vi "Compile Core.vi"(8 "error in (no error)":errorcluster, 10 "Compiled Data":T1 {"DI-B Injection"."Settings"."Pump Phase Array"."Profile" max=15; "DI-B Injection"."Settings"."Pump Phase Array"."Period [s]" min=0 max=0.000102 format="%#_3p"; "DI-B Injection"."Settings"."Pump Phase Array"."Pulse Width [s]" min=0 max=0.000102 format="%#_3p"; "DI-B Injection"."Settings"."Pump Phase Array"."Voltage Low [V]" min=-250 max=250 format="%#_3p"; "DI-B Injection"."Settings"."Pump Phase Array"."Voltage High [V]" min=-250 max=250 format="%#_3p"; "DI-B Injection"."Settings"."Pump Phase Array"."Current Low [A]" min=-40 max=40 format="%#_3p"; "DI-B Injection"."Settings"."Pump Phase Array"."Current High [A]" min=-40 max=40 format="%#_3p"; "DI-B Injection"."Settings"."Pump Phase Array"."Duration [s]" min=0 max=1.67772 format="%#_3p"; "DI-B Injection"."Settings"."Inj Phase Arrays"."Profile" max=15; "DI-B Injection"."Settings"."Inj Phase Arrays"."Period [s]" min=0 max=0.000102 format="%#_3p"; "DI-B Injection"."Settings"."Inj Phase Arrays"."Pulse Width [s]" min=0 max=0.000102 format="%#_3p"; "DI-B Injection"."Settings"."Inj Phase Arrays"."Voltage Low [V]" min=-250 max=250 format="%#_3p"; "DI-B Injection"."Settings"."Inj Phase Arrays"."Voltage High [V]" min=-250 max=250 format="%#_3p"; "DI-B Injection"."Settings"."Inj Phase Arrays"."Current Low [A]" min=-40 max=40 format="%#_3p"; "DI-B Injection"."Settings"."Inj Phase Arrays"."Current High [A]" min=-40 max=40 format="%#_3p"; "DI-B Injection"."Settings"."Inj Phase Arrays"."Duration [s]" min=0 max=1.67772 format="%#_3p"; "DI-A Injection"."Settings"."Pump Phase Array"."Profile" max=15; "DI-A Injection"."Settings"."Pump Phase Array"."Period [s]" min=0 max=0.000102 format="%#_3p"; "DI-A Injection"."Settings"."Pump Phase Array"."Pulse Width [s]" min=0 max=0.000102 format="%#_3p"; "DI-A Injection"."Settings"."Pump Phase Array"."Voltage Low [V]" min=-250 max=250 format="%#_3p"; "DI-A Injection"."Settings"."Pump Phase Array"."Voltage High [V]" min=-250 max=250 format="%#_3p"; "DI-A Injection"."Settings"."Pump Phase Array"."Current Low [A]" min=-40 max=40 format="%#_3p"; "DI-A Injection"."Settings"."Pump Phase Array"."Current High [A]" min=-40 max=40 format="%#_3p"; "DI-A Injection"."Settings"."Pump Phase Array"."Duration [s]" min=0 max=1.67772 format="%#_3p"; "DI-A Injection"."Settings"."Inj Phase Arrays"."Profile" max=15; "DI-A Injection"."Settings"."Inj Phase Arrays"."Period [s]" min=0 max=0.000102 format="%#_3p"; "DI-A Injection"."Settings"."Inj Phase Arrays"."Pulse Width [s]" min=0 max=0.000102 format="%#_3p"; "DI-A Injection"."Settings"."Inj Phase Arrays"."Voltage Low [V]" min=-250 max=250 format="%#_3p"; "DI-A Injection"."Settings"."Inj Phase Arrays"."Voltage High [V]" min=-250 max=250 format="%#_3p"; "DI-A Injection"."Settings"."Inj Phase Arrays"."Current Low [A]" min=-40 max=40 format="%#_3p"; "DI-A Injection"."Settings"."Inj Phase Arrays"."Current High [A]" min=-40 max=40 format="%#_3p"; "DI-A Injection"."Settings"."Inj Phase Arrays"."Duration [s]" min=0 max=1.67772 format="%#_3p"; "Knock"."Settings"."Sensor Select" items=["Sensor 1", "Sensor 2", "Sensor 3", "Sensor 4", "Sensor 5", "Sensor 6", "Sensor 7", "Sensor 8", "Sensor 9", "Sensor 10", "Sensor 11", "Sensor 12"]; "PBx"."PB-01"."FIFO Indexes"."Read"."UEGO Diagnostics"."LSUType" format="%02.0f"; "PBx"."PB-01"."FIFO Indexes"."Read"."UEGO Diagnostics"."UEGOFuseStatus" format="%02.0f"; "DCM Core"."Settings"."System Settings"."HH Open Threshold [A]" min=0 max=8 format="%#_3p"; "DCM Core"."Settings"."System Settings"."HH ISeq Dur PS" items=["3.3ms @ 20MHz"=0, "6.5ms @ 10MHz"=4, "13ms @ 5MHz"=6, "26ms @ 2.5MHz"=7]; "DCM Core"."Settings"."System Settings"."HH Shoot Through Time [s]" min=0 max=0.003277 format="%#_3p"; "DCM Core"."Settings"."System Settings"."Clamp Fault Filter Time [s]" min=0 max=0.003277 format="%#_3p"; "DCM Core"."Settings"."System Settings"."DI HS Fault Filter Time [s]" min=0 max=0.003277 format="%#_3p"; "DCM Core"."Settings"."B Configuration"."Pump Zener Voltage [V]" min=0 max=240 format="%#_13g"; "DCM Core"."Settings"."B Configuration"."DI Zener Voltage [V]" min=0 max=100 format="%#_13g"; "DCM Core"."Settings"."B Configuration"."Boost Clamp [V]" min=0 max=220 format="%#_13g"; "DCM Core"."Settings"."B Configuration"."Boost Voltage [V]" min=0 max=220 format="%#_13g"; "DCM Core"."Settings"."A Configuration"."Pump Zener Voltage [V]" min=0 max=240 format="%#_13g"; "DCM Core"."Settings"."A Configuration"."DI Zener Voltage [V]" min=0 max=100 format="%#_13g"; "DCM Core"."Settings"."A Configuration"."Boost Clamp [V]" min=0 max=220 format="%#_13g"; "DCM Core"."Settings"."A Configuration"."Boost Voltage [V]" min=0 max=220 format="%#_13g"; "DCM Core"."FIFO Indexes"."Write"."HH Config"."ISeq"."Duration [s]" min=0 max=26; "DCM Core"."FIFO Indexes"."Write"."HH Config"."ISeq"."Lower [A]" min=0 max=8; "DCM Core"."FIFO Indexes"."Write"."HH Config"."ISeq"."Upper [A]" min=0 max=8; "Digital Signals"."Settings"."Aux In Filters [s]" min=0; "Digital Signals"."Settings"."Diff IO Filters [s]" min=0; "EPTx RevA"."Settings"."EPTxFilters"."Aux 4 [s]" format="%#_6p"; "EPTx RevA"."Settings"."EPTxFilters"."Aux 3 [s]" format="%#_6p"; "EPTx RevA"."Settings"."EPTxFilters"."Aux 2 [s]" format="%#_6p"; "EPTx RevA"."Settings"."EPTxFilters"."Aux 1 [s]" format="%#_6p"; "EPTx RevA"."Settings"."EPTxFilters"."Primary [s]" format="%#_6p"}, 11 "Device Item Ref in":T40 format="%.0x") -> (0 "error out":errorcluster, 2 "Compiled Data":T1 {"DI-B Injection"."Settings"."Pump Phase Array"."Profile" max=15; "DI-B Injection"."Settings"."Pump Phase Array"."Period [s]" min=0 max=0.000102 format="%#_3p"; "DI-B Injection"."Settings"."Pump Phase Array"."Pulse Width [s]" min=0 max=0.000102 format="%#_3p"; "DI-B Injection"."Settings"."Pump Phase Array"."Voltage Low [V]" min=-250 max=250 format="%#_3p"; "DI-B Injection"."Settings"."Pump Phase Array"."Voltage High [V]" min=-250 max=250 format="%#_3p"; "DI-B Injection"."Settings"."Pump Phase Array"."Current Low [A]" min=-40 max=40 format="%#_3p"; "DI-B Injection"."Settings"."Pump Phase Array"."Current High [A]" min=-40 max=40 format="%#_3p"; "DI-B Injection"."Settings"."Pump Phase Array"."Duration [s]" min=0 max=1.67772 format="%#_3p"; "DI-B Injection"."Settings"."Inj Phase Arrays"."Profile" max=15; "DI-B Injection"."Settings"."Inj Phase Arrays"."Period [s]" min=0 max=0.000102 format="%#_3p"; "DI-B Injection"."Settings"."Inj Phase Arrays"."Pulse Width [s]" min=0 max=0.000102 format="%#_3p"; "DI-B Injection"."Settings"."Inj Phase Arrays"."Voltage Low [V]" min=-250 max=250 format="%#_3p"; "DI-B Injection"."Settings"."Inj Phase Arrays"."Voltage High [V]" min=-250 max=250 format="%#_3p"; "DI-B Injection"."Settings"."Inj Phase Arrays"."Current Low [A]" min=-40 max=40 format="%#_3p"; "DI-B Injection"."Settings"."Inj Phase Arrays"."Current High [A]" min=-40 max=40 format="%#_3p"; "DI-B Injection"."Settings"."Inj Phase Arrays"."Duration [s]" min=0 max=1.67772 format="%#_3p"; "DI-A Injection"."Settings"."Pump Phase Array"."Profile" max=15; "DI-A Injection"."Settings"."Pump Phase Array"."Period [s]" min=0 max=0.000102 format="%#_3p"; "DI-A Injection"."Settings"."Pump Phase Array"."Pulse Width [s]" min=0 max=0.000102 format="%#_3p"; "DI-A Injection"."Settings"."Pump Phase Array"."Voltage Low [V]" min=-250 max=250 format="%#_3p"; "DI-A Injection"."Settings"."Pump Phase Array"."Voltage High [V]" min=-250 max=250 format="%#_3p"; "DI-A Injection"."Settings"."Pump Phase Array"."Current Low [A]" min=-40 max=40 format="%#_3p"; "DI-A Injection"."Settings"."Pump Phase Array"."Current High [A]" min=-40 max=40 format="%#_3p"; "DI-A Injection"."Settings"."Pump Phase Array"."Duration [s]" min=0 max=1.67772 format="%#_3p"; "DI-A Injection"."Settings"."Inj Phase Arrays"."Profile" max=15; "DI-A Injection"."Settings"."Inj Phase Arrays"."Period [s]" min=0 max=0.000102 format="%#_3p"; "DI-A Injection"."Settings"."Inj Phase Arrays"."Pulse Width [s]" min=0 max=0.000102 format="%#_3p"; "DI-A Injection"."Settings"."Inj Phase Arrays"."Voltage Low [V]" min=-250 max=250 format="%#_3p"; "DI-A Injection"."Settings"."Inj Phase Arrays"."Voltage High [V]" min=-250 max=250 format="%#_3p"; "DI-A Injection"."Settings"."Inj Phase Arrays"."Current Low [A]" min=-40 max=40 format="%#_3p"; "DI-A Injection"."Settings"."Inj Phase Arrays"."Current High [A]" min=-40 max=40 format="%#_3p"; "DI-A Injection"."Settings"."Inj Phase Arrays"."Duration [s]" min=0 max=1.67772 format="%#_3p"; "Knock"."Settings"."Sensor Select" items=["Sensor 1", "Sensor 2", "Sensor 3", "Sensor 4", "Sensor 5", "Sensor 6", "Sensor 7", "Sensor 8", "Sensor 9", "Sensor 10", "Sensor 11", "Sensor 12"]; "PBx"."PB-01"."FIFO Indexes"."Read"."UEGO Diagnostics"."LSUType" format="%02.0f"; "PBx"."PB-01"."FIFO Indexes"."Read"."UEGO Diagnostics"."UEGOFuseStatus" format="%02.0f"; "DCM Core"."Settings"."System Settings"."HH Open Threshold [A]" min=0 max=8 format="%#_3p"; "DCM Core"."Settings"."System Settings"."HH ISeq Dur PS" items=["3.3ms @ 20MHz"=0, "6.5ms @ 10MHz"=4, "13ms @ 5MHz"=6, "26ms @ 2.5MHz"=7]; "DCM Core"."Settings"."System Settings"."HH Shoot Through Time [s]" min=0 max=0.003277 format="%#_3p"; "DCM Core"."Settings"."System Settings"."Clamp Fault Filter Time [s]" min=0 max=0.003277 format="%#_3p"; "DCM Core"."Settings"."System Settings"."DI HS Fault Filter Time [s]" min=0 max=0.003277 format="%#_3p"; "DCM Core"."Settings"."B Configuration"."Pump Zener Voltage [V]" min=0 max=240 format="%#_13g"; "DCM Core"."Settings"."B Configuration"."DI Zener Voltage [V]" min=0 max=100 format="%#_13g"; "DCM Core"."Settings"."B Configuration"."Boost Clamp [V]" min=0 max=220 format="%#_13g"; "DCM Core"."Settings"."B Configuration"."Boost Voltage [V]" min=0 max=220 format="%#_13g"; "DCM Core"."Settings"."A Configuration"."Pump Zener Voltage [V]" min=0 max=240 format="%#_13g"; "DCM Core"."Settings"."A Configuration"."DI Zener Voltage [V]" min=0 max=100 format="%#_13g"; "DCM Core"."Settings"."A Configuration"."Boost Clamp [V]" min=0 max=220 format="%#_13g"; "DCM Core"."Settings"."A Configuration"."Boost Voltage [V]" min=0 max=220 format="%#_13g"; "DCM Core"."FIFO Indexes"."Write"."HH Config"."ISeq"."Duration [s]" min=0 max=26; "DCM Core"."FIFO Indexes"."Write"."HH Config"."ISeq"."Lower [A]" min=0 max=8; "DCM Core"."FIFO Indexes"."Write"."HH Config"."ISeq"."Upper [A]" min=0 max=8; "Digital Signals"."Settings"."Aux In Filters [s]" min=0; "Digital Signals"."Settings"."Diff IO Filters [s]" min=0; "EPTx RevA"."Settings"."EPTxFilters"."Aux 4 [s]" format="%#_6p"; "EPTx RevA"."Settings"."EPTxFilters"."Aux 3 [s]" format="%#_6p"; "EPTx RevA"."Settings"."EPTxFilters"."Aux 2 [s]" format="%#_6p"; "EPTx RevA"."Settings"."EPTxFilters"."Aux 1 [s]" format="%#_6p"; "EPTx RevA"."Settings"."EPTxFilters"."Primary [s]" format="%#_6p"}, 3 "Device Item Ref out":T40 format="%.0x")   [LabVIEW 2016, in "DCM System Explorer.lvlib"]
uses:
  DCM System Explorer.lvlib
  <vilib>/NI Veristand/Custom Device API/Custom Device Item Ref.ctl
  Shared/Types/HH Config Indexes.ctl
  Shared/Types/HH Status Indexes.ctl
  Shared/Types/DI Faults Indexes.ctl
  Shared/Types/System State Indexes.ctl
  Shared/Types/Compiled Data.ctl
  <vilib>/NI Veristand/Custom Device Waveform API/Multiple Waveforms Write (DBL)/Multiple Waveforms Write (DBL).lvclass
  Shared/Types/Engine Init Data.ctl
  Shared/Types/Engine Status.ctl
  Shared/Types/EPTx RevA RT Data.ctl
  Built/DCM Classes Packed/Pharlap/C/DCM-Classes.lvlibp/1abvi3w/vi.lib/Powertrain Controls/Device Drivers/DCM/Rev0/FPGA/Digital Channel.ctl
  Built/DCM Classes Packed/Pharlap/C/DCM-Classes.lvlibp/Engine Position Tracking/EPTx/RevA/RT/Controls/EPTxFilters.ctl
  Shared/Types/DCM Core.ctl
  <vilib>/Powertrain Controls/Device Drivers/DCM/Rev0/RT/Configuration.ctl
  <vilib>/Powertrain Controls/Device Drivers/DCM/Rev0/FPGA/DI - Bank Configuration.ctl
  <vilib>/Powertrain Controls/Device Drivers/DCM/Rev0/RT/System Settings.ctl
  <vilib>/Powertrain Controls/Device Drivers/DCM/Rev0/RT/User LED.ctl
  <vilib>/Powertrain Controls/Device Drivers/DCM/HH/RT/Duration Pre Scale.ctl
  Shared/Types/DI.ctl
  Shared/Types/DI Command Indexes.ctl
  Shared/Types/DI Phase Outputs.ctl
  <vilib>/Powertrain Controls/Device Drivers/DCM/DI/RT/Phase.ctl
  <vilib>/Powertrain Controls/Device Drivers/DCM/Rev0/FPGA/DI - Drive State.ctl
  <vilib>/Powertrain Controls/Device Drivers/DCM/DI/FPGA/Phase Step.ctl
  <vilib>/Powertrain Controls/Device Drivers/DCM/DI/FPGA/Control.ctl
  Shared/Types/DiffIO.ctl
  Shared/Types/DiffIO Results Indexes.ctl
  Shared/Types/DiffIO Setup Indexes.ctl
  Shared/Types/HH.ctl
  Shared/Types/HH Command Indexes.ctl
  Shared/Types/DI Scope.ctl
  <vilib>/NI Veristand/Custom Device API/Waveform Data Reference.ctl
  Shared/Types/HH Scope.ctl
  Shared/Types/Digital Signals.ctl
  Shared/Types/Skip Fire.ctl
  Shared/Types/Skip Fire Setup Indexes.ctl
  Shared/Types/Knock.ctl
  Shared/Types/PBx.ctl
  Shared/Types/PB-01.ctl
  Shared/Types/ESTTL Setup Indexes.ctl
  <vilib>/Powertrain Controls/Device Drivers/VR-Hall/RevC/Real-Time/Support/Vr_Hall_mode_control_revc.ctl
  Shared/DCM Properties.vi
  Shared/DCM Constants and GUIDs.vi
  <vilib>/NI Veristand/Custom Device Tools/Custom Device Utility Library/NI VeriStand - Search for Item by GUID.vi
  <vilib>/NI Veristand/Custom Device Tools/Custom Device Utility Library/Custom Device Utility Library.lvlib
  DCM Shared.lvlib
  <vilib>/Powertrain Controls/Device Drivers/DCM/Rev0/RT/DCM - RT.lvclass
  <vilib>/Powertrain Controls/Device Drivers/DCM/HH/RT/DCM - RT - HH.lvlib
  <vilib>/Powertrain Controls/Device Drivers/DCM/Rev0/FPGA/DCM - FPGA.lvlib
  <vilib>/NI VeriStand/Custom Device API/Custom Device API.lvlib
  <vilib>/Powertrain Controls/Device Drivers/DCM/DI/FPGA/DCM - FPGA - DI.lvlib
  <vilib>/Powertrain Controls/Device Drivers/DCM/DI/RT/DCM - RT - DI.lvlib
  Built/DCM Classes Packed/Pharlap/C/DCM-Classes.lvlibp/Engine Position Tracking/EPTx/RevA/RT/EPTx - RevA - RT.lvlib
  Built/DCM Classes Packed/Pharlap/C/DCM-Classes.lvlibp/1abvi3w/vi.lib/Powertrain Controls/Device Drivers/DCM/Rev0/FPGA/DCM - FPGA.lvlib
panel:
  in  "Faults":T9[](array[typedef])=[{"HV Fault"=-1, "LV Fault"=-1, "LS Fault"=-1, "MUX Fault"=-1, "Open Warning"=-1}, {"HV Fault"=-1, "LV Fault"=-1, "LS Fault"=-1, "MUX Fault"=-1, "Open Warning"=-1}, {"HV Fault"=-1, "LV Fault"=-1, "LS Fault"=-1, "MUX Fault"=-1, "Open Warning"=-1}, {"HV Fault"=-1, "LV Fault"=-1, "LS Fault"=-1, "MUX Fault"=-1, "Open Warning"=-1}, {"HV Fault"=-1, "LV Fault"=-1, "LS Fault"=-1, "MUX Fault"=-1, "Open Warning"=-1}, {"HV Fault"=-1, "LV Fault"=-1, "LS Fault"=-1, "MUX Fault"=-1, "Open Warning"=-1}, {"HV Fault"=-1, "LV Fault"=-1, "LS Fault"=-1, "MUX Fault"=-1, "Open Warning"=-1}, {"HV Fault"=-1, "LV Fault"=-1, "LS Fault"=-1, "MUX Fault"=-1, "Open Warning"=-1}]
  in  "Status":T8={"System ADC"={"AI 1 [V]"=-1, "AI 2 [V]"=-1, "AI 3 [V]"=-1, "AI 4 [V]"=-1, "AI 5 [V]"=-1, "AI 6 [V]"=-1, "AI 7 [V]"=-1, "AI 8 [V]"=-1, "AI 9 [V]"=-1, "AI 10 [V]"=-1, "AI 11 [V]"=-1, "AI 12 [V]"=-1, "Temp HH 1-6 [C]"=-1, "Temp HH 7-12 [C]"=-1, "Temp DI A [C]"=-1, "Temp DI Zener A [C]"=-1, "Temp DI B [C]"=-1, "Temp DI Zener B [C]"=-1, "Temp CPU [C]"=-1, "Temp Fan Intake [C]"=-1, "Temp Secondary A [C]"=-1, "Temp Primary A [C]"=-1, "Temp Boost B [C]"=-1, "Primary Range [V]"=-1, "Primary A1A2 [V]"=-1, "Primary A3A4 [V]"=-1, "Primary B3B4 [V]"=-1, "Primary B1B2 [V]"=-1, "Secondary A1A2 [V]"=-1, "Secondary A3A4 [V]"=-1, "Secondary B3B4 [V]"=-1, "Secondary B1B2 [V]"=-1, "Ext HV A [V]"=-1, "Ext HV B [V]"=-1, "FET Driver [V]"=-1, "Fan [V]"=-1, "Battery [V]"=-1, "DRVP [V]"=-1, "Key [V]"=-1, "DI Zener A [V]"=-1, "DI Zener B [V]"=-1, "Pump Zener A [V]"=-1, "Pump Zener B [V]"=-1, "MPRD [V]"=-1}, "IO Lock"=-1, "HH Mode Config Error"=-1, "Fan Speed 1 [RPM]"=-1, "Fan Speed 2 [RPM]"=-1, "Firmware Major Rev"=-1, "Firmware Minor Rev"=-1, "Internal Fault"=-1, "Fault Value"=-1}
  in  "Faults":T9[](array[typedef])=[{"HV Fault"=-1, "LV Fault"=-1, "LS Fault"=-1, "MUX Fault"=-1, "Open Warning"=-1}, {"HV Fault"=-1, "LV Fault"=-1, "LS Fault"=-1, "MUX Fault"=-1, "Open Warning"=-1}, {"HV Fault"=-1, "LV Fault"=-1, "LS Fault"=-1, "MUX Fault"=-1, "Open Warning"=-1}, {"HV Fault"=-1, "LV Fault"=-1, "LS Fault"=-1, "MUX Fault"=-1, "Open Warning"=-1}, {"HV Fault"=-1, "LV Fault"=-1, "LS Fault"=-1, "MUX Fault"=-1, "Open Warning"=-1}, {"HV Fault"=-1, "LV Fault"=-1, "LS Fault"=-1, "MUX Fault"=-1, "Open Warning"=-1}, {"HV Fault"=-1, "LV Fault"=-1, "LS Fault"=-1, "MUX Fault"=-1, "Open Warning"=-1}, {"HV Fault"=-1, "LV Fault"=-1, "LS Fault"=-1, "MUX Fault"=-1, "Open Warning"=-1}]
  in  "Status":T10[](array[typedef])=[{"Current [A]"=-1, "Config Error"=-1, "Short Fault"=-1, "Open Fault"=-1, "Period Min [A]"=-1, "Period Max [A]"=-1, "Period Avg [A]"=-1, "On Avg [A]"=-1}, {"Current [A]"=-1, "Config Error"=-1, "Short Fault"=-1, "Open Fault"=-1, "Period Min [A]"=-1, "Period Max [A]"=-1, "Period Avg [A]"=-1, "On Avg [A]"=-1}, {"Current [A]"=-1, "Config Error"=-1, "Short Fault"=-1, "Open Fault"=-1, "Period Min [A]"=-1, "Period Max [A]"=-1, "Period Avg [A]"=-1, "On Avg [A]"=-1}, {"Current [A]"=-1, "Config Error"=-1, "Short Fault"=-1, "Open Fault"=-1, "Period Min [A]"=-1, "Period Max [A]"=-1, "Period Avg [A]"=-1, "On Avg [A]"=-1}, {"Current [A]"=-1, "Config Error"=-1, "Short Fault"=-1, "Open Fault"=-1, "Period Min [A]"=-1, "Period Max [A]"=-1, "Period Avg [A]"=-1, "On Avg [A]"=-1}, {"Current [A]"=-1, "Config Error"=-1, "Short Fault"=-1, "Open Fault"=-1, "Period Min [A]"=-1, "Period Max [A]"=-1, "Period Avg [A]"=-1, "On Avg [A]"=-1}, {"Current [A]"=-1, "Config Error"=-1, "Short Fault"=-1, "Open Fault"=-1, "Period Min [A]"=-1, "Period Max [A]"=-1, "Period Avg [A]"=-1, "On Avg [A]"=-1}, {"Current [A]"=-1, "Config Error"=-1, "Short Fault"=-1, "Open Fault"=-1, "Period Min [A]"=-1, "Period Max [A]"=-1, "Period Avg [A]"=-1, "On Avg [A]"=-1}, {"Current [A]"=-1, "Config Error"=-1, "Short Fault"=-1, "Open Fault"=-1, "Period Min [A]"=-1, "Period Max [A]"=-1, "Period Avg [A]"=-1, "On Avg [A]"=-1}, {"Current [A]"=-1, "Config Error"=-1, "Short Fault"=-1, "Open Fault"=-1, "Period Min [A]"=-1, "Period Max [A]"=-1, "Period Avg [A]"=-1, "On Avg [A]"=-1}, {"Current [A]"=-1, "Config Error"=-1, "Short Fault"=-1, "Open Fault"=-1, "Period Min [A]"=-1, "Period Max [A]"=-1, "Period Avg [A]"=-1, "On Avg [A]"=-1}, {"Current [A]"=-1, "Config Error"=-1, "Short Fault"=-1, "Open Fault"=-1, "Period Min [A]"=-1, "Period Max [A]"=-1, "Period Avg [A]"=-1, "On Avg [A]"=-1}]
  in  "Config":T11[](array[typedef])=[{"Mode"=-1, "IO Lock State"=-1, "Phase 1 FP"=-1, "Fault Clear"=-1, "ISeq"=[{"Upper [A]"=-1, "Lower [A]"=-1, "Duration [s]"=-1}, {"Upper [A]"=-1, "Lower [A]"=-1, "Duration [s]"=-1}, {"Upper [A]"=-1, "Lower [A]"=-1, "Duration [s]"=-1}, {"Upper [A]"=-1, "Lower [A]"=-1, "Duration [s]"=-1}]}, {"Mode"=-1, "IO Lock State"=-1, "Phase 1 FP"=-1, "Fault Clear"=-1, "ISeq"=[{"Upper [A]"=-1, "Lower [A]"=-1, "Duration [s]"=-1}, {"Upper [A]"=-1, "Lower [A]"=-1, "Duration [s]"=-1}, {"Upper [A]"=-1, "Lower [A]"=-1, "Duration [s]"=-1}, {"Upper [A]"=-1, "Lower [A]"=-1, "Duration [s]"=-1}]}, {"Mode"=-1, "IO Lock State"=-1, "Phase 1 FP"=-1, "Fault Clear"=-1, "ISeq"=[{"Upper [A]"=-1, "Lower [A]"=-1, "Duration [s]"=-1}, {"Upper [A]"=-1, "Lower [A]"=-1, "Duration [s]"=-1}, {"Upper [A]"=-1, "Lower [A]"=-1, "Duration [s]"=-1}, {"Upper [A]"=-1, "Lower [A]"=-1, "Duration [s]"=-1}]}, {"Mode"=-1, "IO Lock State"=-1, "Phase 1 FP"=-1, "Fault Clear"=-1, "ISeq"=[{"Upper [A]"=-1, "Lower [A]"=-1, "Duration [s]"=-1}, {"Upper [A]"=-1, "Lower [A]"=-1, "Duration [s]"=-1}, {"Upper [A]"=-1, "Lower [A]"=-1, "Duration [s]"=-1}, {"Upper [A]"=-1, "Lower [A]"=-1, "Duration [s]"=-1}]}, {"Mode"=-1, "IO Lock State"=-1, "Phase 1 FP"=-1, "Fault Clear"=-1, "ISeq"=[{"Upper [A]"=-1, "Lower [A]"=-1, "Duration [s]"=-1}, {"Upper [A]"=-1, "Lower [A]"=-1, "Duration [s]"=-1}, {"Upper [A]"=-1, "Lower [A]"=-1, "Duration [s]"=-1}, {"Upper [A]"=-1, "Lower [A]"=-1, "Duration [s]"=-1}]}, {"Mode"=-1, "IO Lock State"=-1, "Phase 1 FP"=-1, "Fault Clear"=-1, "ISeq"=[{"Upper [A]"=-1, "Lower [A]"=-1, "Duration [s]"=-1}, {"Upper [A]"=-1, "Lower [A]"=-1, "Duration [s]"=-1}, {"Upper [A]"=-1, "Lower [A]"=-1, "Duration [s]"=-1}, {"Upper [A]"=-1, "Lower [A]"=-1, "Duration [s]"=-1}]}, {"Mode"=-1, "IO Lock State"=-1, "Phase 1 FP"=-1, "Fault Clear"=-1, "ISeq"=[{"Upper [A]"=-1, "Lower [A]"=-1, "Duration [s]"=-1}, {"Upper [A]"=-1, "Lower [A]"=-1, "Duration [s]"=-1}, {"Upper [A]"=-1, "Lower [A]"=-1, "Duration [s]"=-1}, {"Upper [A]"=-1, "Lower [A]"=-1, "Duration [s]"=-1}]}, {"Mode"=-1, "IO Lock State"=-1, "Phase 1 FP"=-1, "Fault Clear"=-1, "ISeq"=[{"Upper [A]"=-1, "Lower [A]"=-1, "Duration [s]"=-1}, {"Upper [A]"=-1, "Lower [A]"=-1, "Duration [s]"=-1}, {"Upper [A]"=-1, "Lower [A]"=-1, "Duration [s]"=-1}, {"Upper [A]"=-1, "Lower [A]"=-1, "Duration [s]"=-1}]}, {"Mode"=-1, "IO Lock State"=-1, "Phase 1 FP"=-1, "Fault Clear"=-1, "ISeq"=[{"Upper [A]"=-1, "Lower [A]"=-1, "Duration [s]"=-1}, {"Upper [A]"=-1, "Lower [A]"=-1, "Duration [s]"=-1}, {"Upper [A]"=-1, "Lower [A]"=-1, "Duration [s]"=-1}, {"Upper [A]"=-1, "Lower [A]"=-1, "Duration [s]"=-1}]}, {"Mode"=-1, "IO Lock State"=-1, "Phase 1 FP"=-1, "Fault Clear"=-1, "ISeq"=[{"Upper [A]"=-1, "Lower [A]"=-1, "Duration [s]"=-1}, {"Upper [A]"=-1, "Lower [A]"=-1, "Duration [s]"=-1}, {"Upper [A]"=-1, "Lower [A]"=-1, "Duration [s]"=-1}, {"Upper [A]"=-1, "Lower [A]"=-1, "Duration [s]"=-1}]}, {"Mode"=-1, "IO Lock State"=-1, "Phase 1 FP"=-1, "Fault Clear"=-1, "ISeq"=[{"Upper [A]"=-1, "Lower [A]"=-1, "Duration [s]"=-1}, {"Upper [A]"=-1, "Lower [A]"=-1, "Duration [s]"=-1}, {"Upper [A]"=-1, "Lower [A]"=-1, "Duration [s]"=-1}, {"Upper [A]"=-1, "Lower [A]"=-1, "Duration [s]"=-1}]}, {"Mode"=-1, "IO Lock State"=-1, "Phase 1 FP"=-1, "Fault Clear"=-1, "ISeq"=[{"Upper [A]"=-1, "Lower [A]"=-1, "Duration [s]"=-1}, {"Upper [A]"=-1, "Lower [A]"=-1, "Duration [s]"=-1}, {"Upper [A]"=-1, "Lower [A]"=-1, "Duration [s]"=-1}, {"Upper [A]"=-1, "Lower [A]"=-1, "Duration [s]"=-1}]}] {"ISeq"."Duration [s]" min=0 max=26; "ISeq"."Lower [A]" min=0 max=8; "ISeq"."Upper [A]" min=0 max=8}
  # "DI-A"
  # "DI-B"
  # "Voltage [DV]"
  # "Voltage [V]"
  # "Voltage [DV]"
  # "Voltage [V]"
  # "Voltage [DV]"
  # "Voltage [V]"
  # "Voltage [DV]"
  # "Voltage [V]"
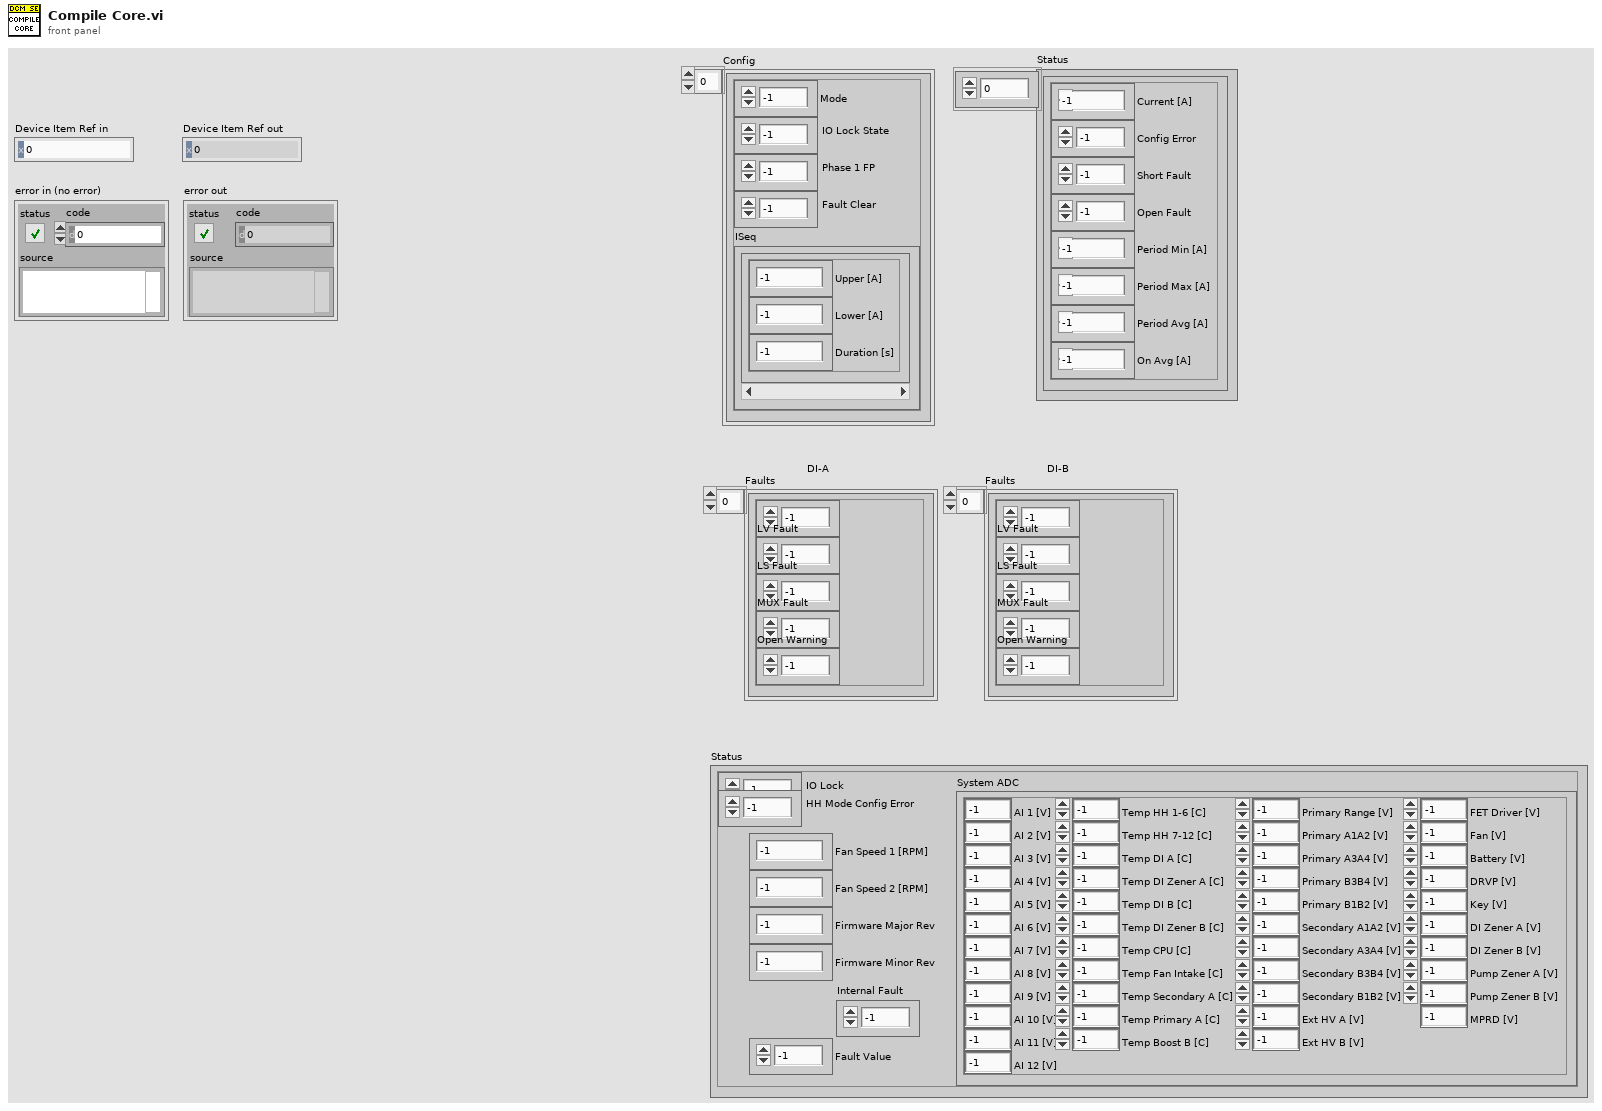
[diagram p1: front panel]
types:
  T1 = typedef "DCM Shared.lvlib/Compiled Data.ctl" = cluster{"Init":T2, "Cmd Status":T3, "Sys Status":T3, "EPTx RevA":T4, "DCM Core":T7, "DI-A Injection":T17, "DI-B Injection":T17, "DiffIO":T24, "HH Cmd":T27, "DI ADC":T29, "HH ADC":T31, "Digital Signals":T32, "Skip Fire":T33, "Knock":T35, "PBx":T36}
  T2 = typedef "DCM Shared.lvlib/Engine Init Data.ctl" = cluster{"Name":string, "RIO Address":string, "Bitfile Path RT":path, "Username":string, "Password":string, "Cmd CPU":i32, "Cmd Decimation":i32, "Cmd Priority":i32, "Sys CPU":i32, "Sys Decimation":i32, "Sys Priority":i32, "Input FIFO Size":i32, "Output FIFO Size":i32, "Compile Time":dbl}
  T3 = typedef "DCM Shared.lvlib/Engine Status.ctl" = cluster{"FIFO indexes":cluster{"code":i32, "loop duration":i32, "late count":i32}}
  T4 = typedef "DCM Shared.lvlib/EPTx RevA RT Data.ctl" = cluster{"FIFO Indexes":cluster{"Read":cluster{"Sync":i32, "CurrentCAD":i32, "Speed":i32, "Config":i32, "Rcvg Primary":i32, "Stall":i32, "Overflow Error":i32, "Ratio Error":i32, "Pattern Error":i32, "Aux Warning":i32, "Watchdog Error":i32, "Loading":i32}, "Write":cluster{"Reload EPTx":i32, "Sync Enable":i32, "Clear Errors":i32, "Sim Enable":i32, "Sim Speed":i32}}, "Settings":cluster{"EPTxConfigFilename":string, "EPTx Signal Select":cluster{"Primary":T5, "Aux 1":T5, "Aux 2":T5, "Aux 3":T5, "Aux 4":T5}, "FPGAFrequency":sgl, "StallSpeed":sgl, "EPTxFilters":T6, "History":u8}}
  T5 = typedef "DCM-Classes.lvlibp/DCM - FPGA.lvlib/Digital Channel.ctl" = enum8{"Unused", "User OS", "Diff IO 1", "Diff IO 2", "Diff IO 3", "Diff IO 4", "Diff IO 5", "Diff IO 6", "Diff IO 7", "Diff IO 8", "Aux 1", "Aux 2", "Aux 3", "Aux 4", "Aux 5", "Aux 6", "Aux 7", "Aux 8", "Aux 9", "Aux 10", "Aux 11", "Aux 12", "Aux 13", "Aux 14", "Aux 15", "Aux 16"}
  T6 = typedef "DCM-Classes.lvlibp/EPTx - RevA - RT.lvlib/EPTxFilters.ctl" = cluster{"Primary [s]":sgl, "Aux 1 [s]":sgl, "Aux 2 [s]":sgl, "Aux 3 [s]":sgl, "Aux 4 [s]":sgl}
  T7 = typedef "DCM Shared.lvlib/DCM Core.ctl" = cluster{"FIFO Indexes":cluster{"A Run State":i32, "B Run State":i32, "Read":cluster{"Status":T8, "A DI Faults":T9[], "B DI Faults":T9[], "HH Status":T10[]}, "Write":cluster{"A Config":cluster{"PowerSupplyEnable":i32, "InjectEnable":i32, "BoostVoltage":i32}, "B Config":cluster{"PowerSupplyEnable":i32, "InjectEnable":i32, "BoostVoltage":i32}, "HH Config":T11[], "System Settings":cluster{"MPRD":i32, "UserLED1":i32, "UserLED2":i32}, "A Fault Clear":cluster{"1":i32, "2":i32, "3":i32, "4":i32, "5":i32, "6":i32, "7":i32, "8":i32}, "B Fault Clear":cluster{"1":i32, "2":i32, "3":i32, "4":i32, "5":i32, "6":i32, "7":i32, "8":i32}}}, "Settings":cluster{"A Configuration":T12, "B Configuration":T12, "System Settings":T14}}
  T8 = typedef "DCM Shared.lvlib/System State Indexes.ctl" = cluster{"System ADC":cluster{"AI 1 [V]":i32, "AI 2 [V]":i32, "AI 3 [V]":i32, "AI 4 [V]":i32, "AI 5 [V]":i32, "AI 6 [V]":i32, "AI 7 [V]":i32, "AI 8 [V]":i32, "AI 9 [V]":i32, "AI 10 [V]":i32, "AI 11 [V]":i32, "AI 12 [V]":i32, "Temp HH 1-6 [C]":i32, "Temp HH 7-12 [C]":i32, "Temp DI A [C]":i32, "Temp DI Zener A [C]":i32, "Temp DI B [C]":i32, "Temp DI Zener B [C]":i32, "Temp CPU [C]":i32, "Temp Fan Intake [C]":i32, "Temp Secondary A [C]":i32, "Temp Primary A [C]":i32, "Temp Boost B [C]":i32, "Primary Range [V]":i32, "Primary A1A2 [V]":i32, "Primary A3A4 [V]":i32, "Primary B3B4 [V]":i32, "Primary B1B2 [V]":i32, "Secondary A1A2 [V]":i32, "Secondary A3A4 [V]":i32, "Secondary B3B4 [V]":i32, "Secondary B1B2 [V]":i32, "Ext HV A [V]":i32, "Ext HV B [V]":i32, "FET Driver [V]":i32, "Fan [V]":i32, "Battery [V]":i32, "DRVP [V]":i32, "Key [V]":i32, "DI Zener A [V]":i32, "DI Zener B [V]":i32, "Pump Zener A [V]":i32, "Pump Zener B [V]":i32, "MPRD [V]":i32}, "IO Lock":i32, "HH Mode Config Error":i32, "Fan Speed 1 [RPM]":i32, "Fan Speed 2 [RPM]":i32, "Firmware Major Rev":i32, "Firmware Minor Rev":i32, "Internal Fault":i32, "Fault Value":i32}
  T9 = typedef "DCM Shared.lvlib/DI Faults Indexes.ctl" = cluster{"HV Fault":i32, "LV Fault":i32, "LS Fault":i32, "MUX Fault":i32, "Open Warning":i32}
  T10 = typedef "DCM Shared.lvlib/HH Status Indexes.ctl" = cluster{"Current [A]":i32, "Config Error":i32, "Short Fault":i32, "Open Fault":i32, "Period Min [A]":i32, "Period Max [A]":i32, "Period Avg [A]":i32, "On Avg [A]":i32}
  T11 = typedef "DCM Shared.lvlib/HH Config Indexes.ctl" = cluster{"Mode":i32, "IO Lock State":i32, "Phase 1 FP":i32, "Fault Clear":i32, "ISeq":cluster{"Upper [A]":i32, "Lower [A]":i32, "Duration [s]":i32}[]}
  T12 = typedef "DCM - RT.lvclass/Configuration.ctl" = cluster{"Configuration":T13, "Power Supply Enable":bool, "Boost Voltage [V]":sgl, "Inject Enable":bool, "DI Zener Enable":bool, "DI Zener Voltage [V]":sgl, "Pump Zener Enable":bool, "Pump Zener Voltage [V]":sgl, "Boost Clamp [V]":sgl}
  T13 = typedef "DCM - FPGA.lvlib/DI - Bank Configuration.ctl" = enum8{"Solenoid Unipolar 4", "Solenoid Unipolar 7 (Muxed)", "Solenoid Unipolar 8 (Muxed)", "Solenoid Bipolar 2", "Solenoid Bipolar 3 (Muxed)", "Piezo Unipolar 2", "Piezo Unipolar 3 (Muxed)", "Piezo Unipolar 4 (Muxed)", "Piezo Bipolar 2", "Piezo Bipolar 3 (Muxed)"}
  T14 = typedef "DCM - RT.lvclass/System Settings.ctl" = cluster{"MPRD":bool, "IO Lock MPRD Disable":bool, "User LED 1":T15, "User LED 2":T15, "DI HS Fault Filter Time [s]":sgl, "Clamp Fault Filter Time [s]":sgl, "HH Shoot Through Time [s]":sgl, "HH ISeq Dur PS":T16, "HH Open Threshold [A]":sgl}
  T15 = typedef "DCM - RT.lvclass/User LED.ctl" = enum16{"Off", "Yellow", "Green"}
  T16 = typedef "DCM - RT - HH.lvlib/Duration Pre Scale.ctl" = u8
  T17 = typedef "DCM Shared.lvlib/DI.ctl" = cluster{"DI Command Enabled":bool, "Sync Pump Enabled":bool, "FIFO Indexes":cluster{"Write":cluster{"DI Command":T18[], "Pump Command":T18}}, "Settings":T19}
  T18 = typedef "DCM Shared.lvlib/DI Command Indexes.ctl" = cluster{"Mode":i32, "Digital Input":i32, "Default Profile Index":i32, "Cal Freq [Hz]":i32, "Cal Duration [s]":i32, "Cal Increment [s]":i32, "Cal Pulses":i32, "TMP Command Sequence":cluster{"Duration [s]":i32, "Level":i32, "Run/Stop":i32, "Profile Index":i32}[], "EPT TDC Offset [CAD]":i32, "EPT Window Start [DBTDC]":i32, "EPT Window End [DBTDC]":i32, "EPT Angles":cluster{"Enable":i32, "Timing [DBTDC]":i32, "Duration [s]":i32, "Profile Index":i32}[], "EPT Skip Fire":i32, "EPT Skip Index":i32, "EPT Precharge Duration [s]":i32, "EPT Precharge Profile Index":i32}
  T19 = typedef "DCM Shared.lvlib/DI Phase Outputs.ctl" = cluster{"Inj Phase Arrays":T20[][], "Pump Phase Array":T20[], "Pulsewidths [s]":sgl[][]}
  T20 = typedef "DCM - RT - DI.lvlib/Phase.ctl" = cluster{"Drive":T21, "Direction":bool, "Phase Step":T22, "Duration [s]":sgl, "Current High [A]":sgl, "Current Low [A]":sgl, "Voltage High [V]":sgl, "Voltage Low [V]":sgl, "Change":bool, "Current Control":T23, "Period [s]":sgl, "Pulse Width [s]":sgl, "Profile":u8, "Voltage Control":bool}
  T21 = typedef "DCM - FPGA.lvlib/DI - Drive State.ctl" = enum8{"Idle", "HV Current Control", "LV Current Control", "Back Boost", "Piezo Charge", "Piezo Discharge"}
  T22 = typedef "DCM - FPGA - DI.lvlib/Phase Step.ctl" = enum8{"Duration", "First Peak", "End of Cmd", "Branch", "2-Phase Duration"}
  T23 = typedef "DCM - FPGA - DI.lvlib/Control.ctl" = enum8{"Closed Loop", "Fixed Period", "Fixed On Pulse", "Fixed Off Pulse", "Open Loop", "Profile"}
  T24 = typedef "DCM Shared.lvlib/DiffIO.ctl" = cluster{"DiffIO Command Enabled":bool, "FIFO Indexes":cluster{"Read":cluster{"Diff IO Results":T25[], "DiffIOIn":cluster{"1":i32, "2":i32, "3":i32, "4":i32, "5":i32, "6":i32, "7":i32, "8":i32}}, "Write":cluster{"Diff I/O Setup":T26[]}}}
  T25 = typedef "DCM Shared.lvlib/DiffIO Results Indexes.ctl" = cluster{"Capture [DBTDC]":i32, "Capture Error":i32, "Frequency [Hz]":i32, "Duty Cycle [%]":i32, "PWM Stopped":i32}
  T26 = typedef "DCM Shared.lvlib/DiffIO Setup Indexes.ctl" = cluster{"Mode":i32, "Capture Start [DBTDC]":i32, "Capture End [DBTDC]":i32, "Polarity":i32, "Frequency [Hz]":i32, "Duty Cycle [%]":i32, "TDC Offset [CAD]":i32, "Window Start [DBTDC]":i32, "Window End [DBTDC]":i32, "Angles":cluster{"Enable":i32, "Location [DBTDC]":i32, "Duration [s]":i32}[], "Skip Fire":i32, "Skip Fire Index":i32}
  T27 = typedef "DCM Shared.lvlib/HH.ctl" = cluster{"HH Command Enabled":bool, "FIFO Indexes":cluster{"Write":T28[]}}
  T28 = typedef "DCM Shared.lvlib/HH Command Indexes.ctl" = cluster{"Mode":i32, "Digital Input":i32, "Polarity":i32, "Frequency [Hz]":i32, "Duty Cycle [%]":i32, "TDC Offset [CAD]":i32, "Window Start [DBTDC]":i32, "Window End [DBTDC]":i32, "Angles":cluster{"Enable":i32, "Location [DBTDC]":i32, "Duration [s]":i32}[], "Skip Fire":i32, "Skip Fire Index":i32}
  T29 = typedef "DCM Shared.lvlib/DI Scope.ctl" = cluster{"FIFO Indexes":cluster{"Write":cluster{"Capture Enable":i32, "Capture Event":i32, "Capture Length":i32, "DI ADC 1 Select":i32, "DI ADC 2 Select":i32, "DI ADC 3 Select":i32, "DI ADC 4 Select":i32}, "Read":cluster{"Capture dt [s]":i32}}, "DI ADC Data":cluster{"Output Array":sgl[][], "New Data":bool}, "Waveform Data":T30[], "Waveform Session":refnum<class "Multiple Waveforms Write (DBL).lvclass">}
  T30 = typedef "Custom Device API.lvlib/Waveform Data Reference.ctl" = i32
  T31 = typedef "DCM Shared.lvlib/HH Scope.ctl" = cluster{"FIFO Indexes":cluster{"Write":cluster{"Capture Enable":i32, "Capture Event":i32, "Capture Length":i32}, "Read":cluster{"Capture dt [s]":i32}}, "HH ADC Data":cluster{"Output Array":sgl[][], "New Data":bool}, "Waveform Data":T30[], "Waveform Session":refnum<class "Multiple Waveforms Write (DBL).lvclass">}
  T32 = typedef "DCM Shared.lvlib/Digital Signals.ctl" = cluster{"FIFO Indexes":cluster{"Write":cluster{"User OS":i32, "User OS Time [s]":i32}}, "Settings":cluster{"Diff IO Filters [s]":sgl[], "Aux In Filters [s]":sgl[]}}
  T33 = typedef "DCM Shared.lvlib/Skip Fire.ctl" = cluster{"Skip Fire Enabled":bool, "FIFO Indexes":cluster{"Write":cluster{"Setup":T34[]}}}
  T34 = typedef "DCM Shared.lvlib/Skip Fire Setup Indexes.ctl" = cluster{"Enable":i32, "Total Cycles":i32, "On Cycles":i32, "TDC Offset [CAD]":i32}
  T35 = typedef "DCM Shared.lvlib/Knock.ctl" = cluster{"FIFO Indexes":cluster{"Read":cluster{"Knock":i32[], "Knock Intensity":i32[]}, "Write":cluster{"Low Cutoff [Hz]":i32, "High Cutoff [Hz]":i32, "Threshold":i32, "Knock Start [CAD]":i32, "Knock End [CAD]":i32, "Reference Start [CAD]":i32, "Reference End [CAD]":i32}}, "Settings":cluster{"Sensor Select":i32[], "Cylinder Offset [CAD]":sgl[]}}
  T36 = typedef "DCM Shared.lvlib/PBx.ctl" = cluster{"PB Version":u8, "PB-01":T37}
  T37 = typedef "DCM Shared.lvlib/PB-01.ctl" = cluster{"FIFO Indexes":cluster{"Write":cluster{"Clear Faults":i32, "ESTTL Setup":T38[], "UEGO Control":cluster{"UEGO1Enable":i32, "UEGO2Enable":i32, "UEGO1Range":i32, "UEGO2Range":i32, "FilterCutoff (Hz)":i32}}, "Read":cluster{"UEGO Sensor Results":cluster{"UEGO1Lambda":i32, "UEGO1Phi":i32, "UEGO1AFRatio":i32, "UEGO1Ip (mA)":i32, "UEGO2Lambda":i32, "UEGO2Phi":i32, "UEGO2AFRatio":i32, "UEGO2Ip (mA)":i32}, "UEGO Temperature (C)":cluster{"UEGO1Temp (C)":i32, "UEGO2Temp (C)":i32, "UEGO1Hot":i32, "UEGO2Hot":i32}, "UEGO Diagnostics":cluster{"UEGO1SensorFault":i32, "UEGO2SensorFault":i32, "UEGO1HeaterFault":i32, "UEGO2HeaterFault":i32, "UEGOFuseStatus":i32, "Battery (V)":i32, "LSUType":i32}}}, "Settings":cluster{"VR-Hall Mode Select":T39[], "VR-Hall Arming Threshold [V]":dbl[], "ESTTL Command Enabled":bool}}
  T38 = typedef "DCM Shared.lvlib/ESTTL Setup Indexes.ctl" = cluster{"Mode":i32, "Polarity":i32, "Frequency [Hz]":i32, "Duty Cycle [%]":i32, "TDC Offset [CAD]":i32, "Window Start [DBTDC]":i32, "Window End [DBTDC]":i32, "Angles":cluster{"Enable":i32, "Location [DBTDC]":i32, "Duration [s]":i32}[], "Skip Fire":i32, "Skip Fire Index":i32}
  T39 = typedef "Vr_Hall_mode_control_revc.ctl" = enum32{"VR Adaptive Arm", "VR Manual Arm", "Hall", "Hall w/ Pull-up"}
  T40 = typedef "Custom Device API.lvlib/Custom Device Item Ref.ctl" = u64
  T41 = typedef "DCM Shared.lvlib/Channel.ctl" = cluster{"Name":string, "Units":string, "Default":dbl, "Description":string}
  T42 = cluster{"FIFO indexes[0]":i32, "FIFO indexes[1]":i32, "FIFO indexes[2]":i32}
  T43 = cluster{"FIFO indexes[0]":i32, "FIFO indexes[1]":i32, "FIFO indexes[2]":i32, "FIFO indexes[3]":i32, "FIFO indexes[4]":i32, "FIFO indexes[5]":i32, "FIFO indexes[6]":i32, "FIFO indexes[7]":i32}
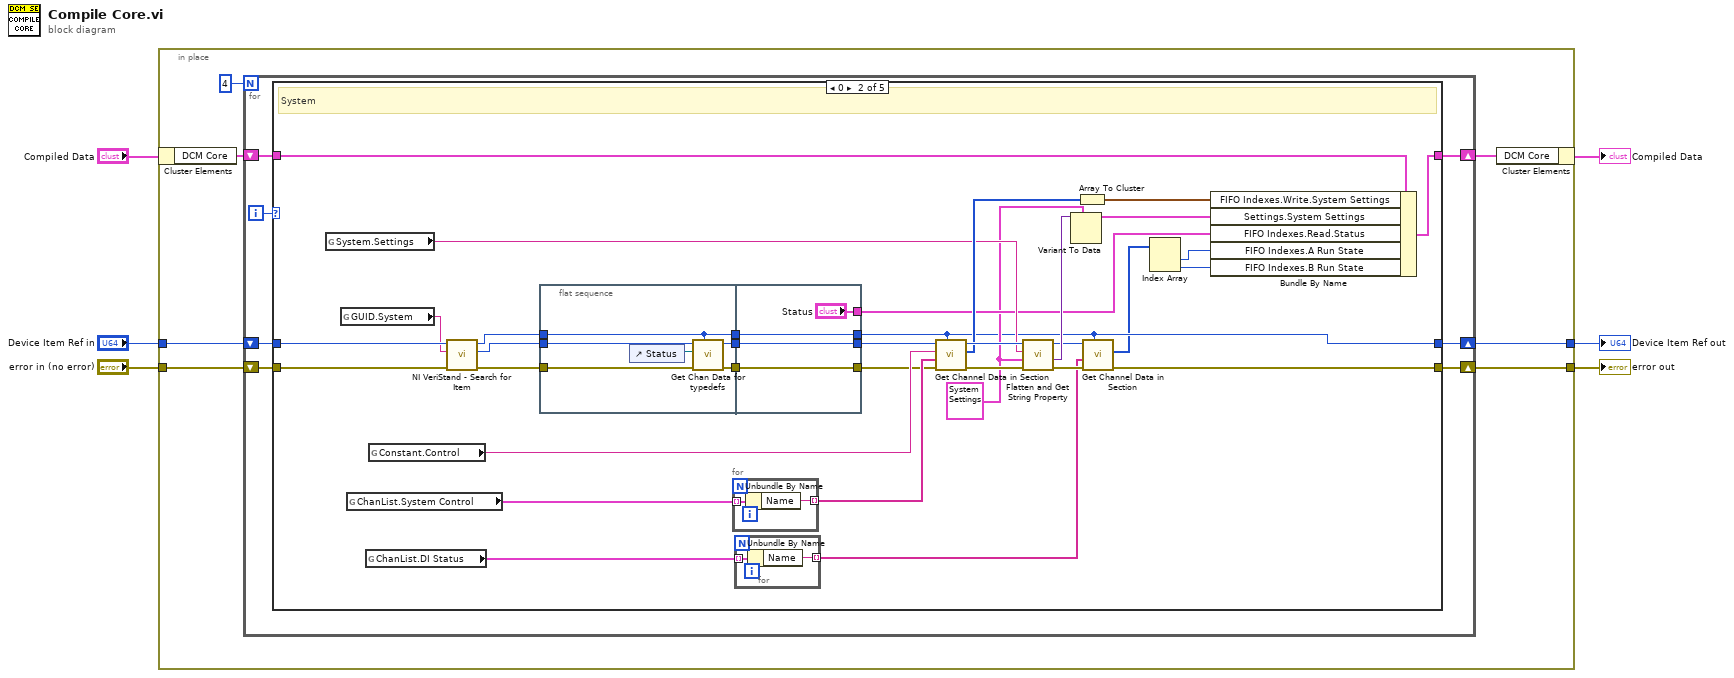
[diagram p0: block diagram]
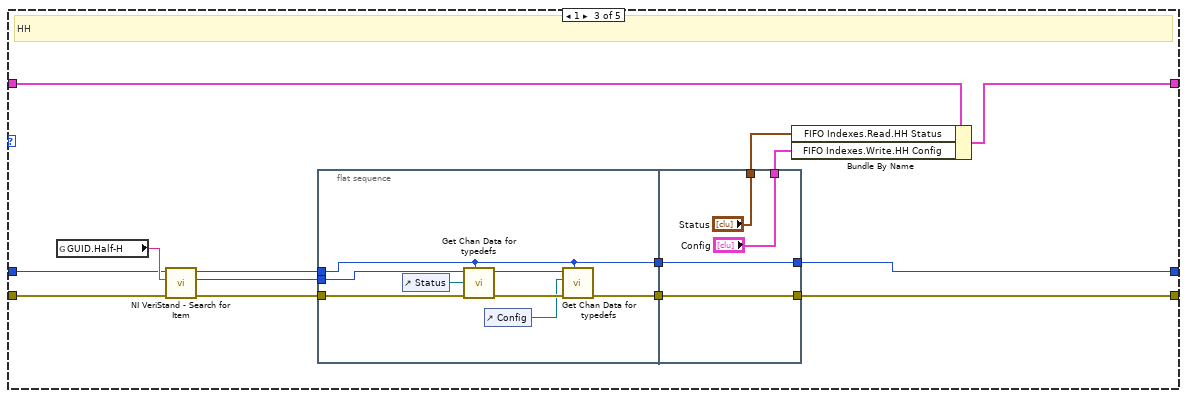
[diagram p3: hidden frame]
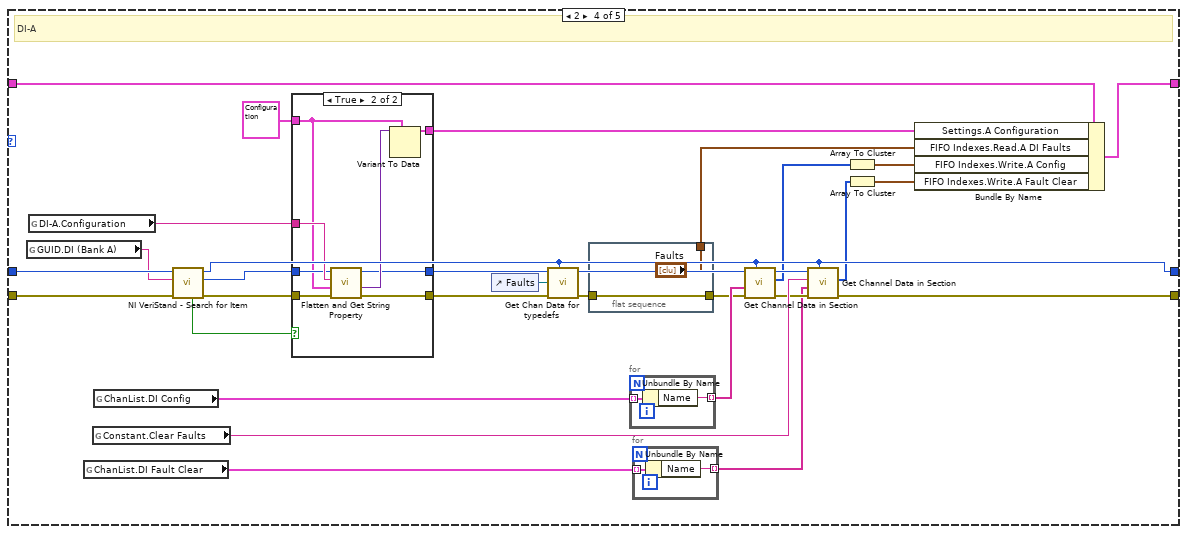
[diagram p4: hidden frame]
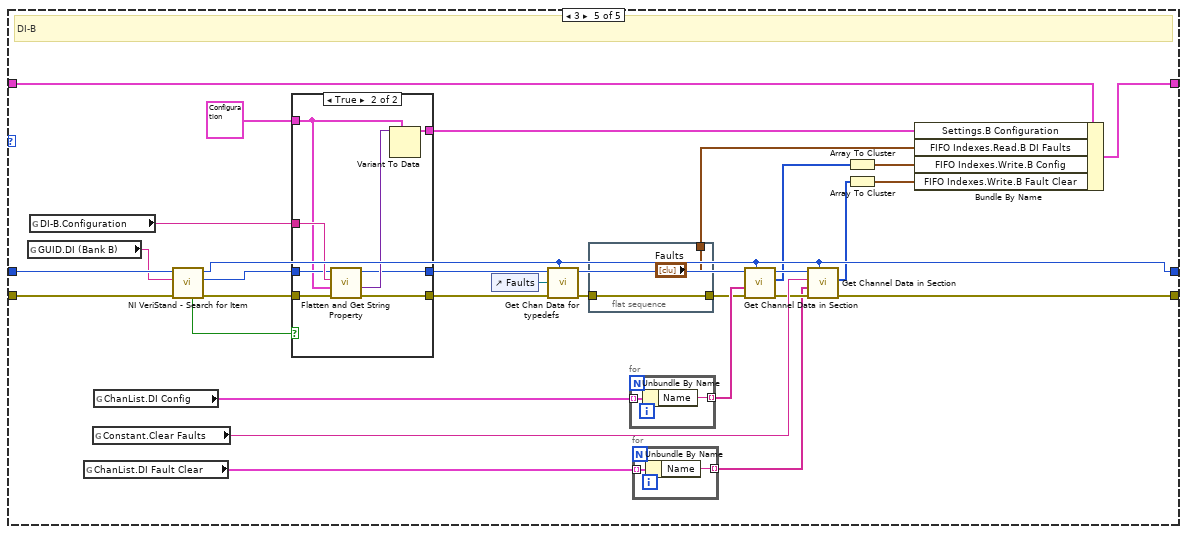
[diagram p6: hidden frame]
diagram:
  n1 = in-place {
    in-place-border: "error in (no error)" -> [w13]
    in-place-border: "Device Item Ref in" -> [w12]
    in-place-border: [w11] -> w4
    in-place-border: [w9] -> w3
    n2 = in-place-cluster #1("Compiled Data") -> ("DCM Core"=w8:T7)
    n3 = for {
      N: 4 -> [_]
      shift-right: [w18] -> w9
      shift-left: w13 -> [w20]
      shift-right: [w14] -> w11
      shift-left: w12 -> [w19]
      shift-right: [w15] -> w7
      shift-left: w8 -> [w16]
      i -> [w17]
      n4 = case shown="0" w17 {
        tunnel: w20 -> [w22 w57 w79 w128 w176]
        tunnel: w19 -> [w23 w56 w80 w127 w175]
        tunnel: [w22 w29 w82 w122 w170] -> w18
        tunnel: w16 -> [w21 w45 w85 w121 w169]
        tunnel: [w21 w44 w84 w120 w168] -> w15
        tunnel: [w23 w28 w83 w118 w166] -> w14
        frame -1, Default {
        }
        frame 0 {
          w33 = T14 {"MPRD"=FALSE, "IO Lock MPRD Disable"=FALSE, "User LED 1"=enum."Off", "User LED 2"=enum."Off", "DI HS Fault Filter Time [s]"=0.0, "Clamp Fault Filter Time [s]"=0.0, "HH Shoot Through Time [s]"=0.0, "HH ISeq Dur PS"=0, "HH Open Threshold [A]"=0.1} ("outputs.System Settings")
          # "System"
          n5 = global read "DCM Properties.vi" "System.Settings"() -> (w47:string)
          n6 = global read "DCM Constants and GUIDs.vi" "GUID.System"() -> (w55:string)
          n7 = global read "DCM Constants and GUIDs.vi" "ChanList.System Control"() -> (w53:T41[])
          n8 = global read "DCM Constants and GUIDs.vi" "ChanList.DI Status"() -> (w32:T41[])
          n9 = global read "DCM Constants and GUIDs.vi" "Constant.Control"() -> (w48:string)
          n10 = call-poly <vilib>:"NI VeriStand - Search for Item.vi"("error in"=w57, "Item GUID"=w55, "Section Ref in"=w56) -> ("error out"=w42:errorcluster, "Item Ref"=w43:T40, "Section Ref out"=w39:T40)  [unwired: 5 in, 1 out]
          n11 = flat-sequence {
            tunnel: w43 -> [w65]
            tunnel: w42 -> [w63]
            tunnel: [w64] -> w41
            tunnel: [w62] -> w40
            tunnel: w39 -> [w61]
            tunnel: [w61] -> w38
            tunnel: [w68] -> w34
            tunnel: [w69] -> w35
            tunnel: w41 -> [w69]
            tunnel: w40 -> [w68]
            tunnel: ["Status"] -> w37
            tunnel: [w67] -> w28
            tunnel: w38 -> [w67]
            frame #0 {
              n12 = control-ref of="Status"() -> (w60:refnum<vi>)
              n13 = call "Get Chan Data for typedefs.vi"("Custom Device Ref"=w61, "error in"=w63, "Ctl Ref"=w60, "Section Ref in"=w65) -> ("error out"=w62:errorcluster, "Section Ref out"=w64:T40)  [unwired: 5 in, 1 out]
            }
            frame #1 {
            }
          }
          n14 = for {
            tunnel: w53 -> [w71] mode=indexing
            tunnel: [w70] -> w49 mode=indexing
            n15 = Unbundle By Name(w71) -> ("Name"=w70:string)
          }
          n16 = for {
            tunnel: w32 -> [w59] mode=indexing
            tunnel: [w58] -> w27 mode=indexing
            n17 = Unbundle By Name(w59) -> ("Name"=w58:string)
          }
          n18 = call "Get Channel Data in Section.vi"("Custom device ref"=w28, "error in (no error)"=w34, "Channels"=w49, "Section (\"\":none)"=w48, "Item Ref in"=w35) -> ("error out"=w52:errorcluster, "FIFO indexes"=w50:i32[], "Item Ref out"=w51:T40)  [unwired: 2 in, 2 out]
          n19 = call "Flatten and Get String Property.vi"("error in (no error)"=w52, "Default Value"=w33, "Property Name"=w47, "Section Ref in"=w51) -> ("error out"=w30:errorcluster, "Value"=w54:variant, "Section Ref out"=w31:T40)  [unwired: 5 in]
          n20 = Variant To Data(type=w33, Variant=w54) -> (data=w36:T14)  [unwired: 1 in, 1 out]
          n21 = Array To Cluster(array=w50) -> (cluster=w46:T42)
          n22 = call "Get Channel Data in Section.vi"("Custom device ref"=w28, "error in (no error)"=w30, "Channels"=w27, "Item Ref in"=w31) -> ("error out"=w29:errorcluster, "FIFO indexes"=w26:i32[])  [unwired: 3 in, 3 out]
          n23 = Index Array(array=w26) -> (element #1=w25:i32, element #2=w24:i32)  [unwired: 2 in]
          n24 = Bundle By Name(cluster=w45, "FIFO Indexes.Write.System Settings"=w46, "Settings.System Settings"=w36, "FIFO Indexes.Read.Status"=w37, "FIFO Indexes.A Run State"=w25, "FIFO Indexes.B Run State"=w24) -> (w44:T7)
        }
        frame 1 {
          # "HH"
          n25 = global read "DCM Constants and GUIDs.vi" "GUID.Half-H"() -> (w81:string)
          n26 = call-poly <vilib>:"NI VeriStand - Search for Item.vi"("error in"=w79, "Item GUID"=w81, "Section Ref in"=w80) -> ("error out"=w77:errorcluster, "Item Ref"=w78:T40, "Section Ref out"=w76:T40)  [unwired: 5 in, 1 out]
          n27 = flat-sequence {
            tunnel: [w86] -> w75
            tunnel: [w93] -> w74
            tunnel: w78 -> [w88]
            tunnel: w77 -> [w87]
            tunnel: w76 -> [w86]
            tunnel: [w96] -> w82
            tunnel: [w97] -> w83
            tunnel: w75 -> [w97]
            tunnel: w74 -> [w96]
            tunnel: ["Status"] -> w73
            tunnel: ["Config"] -> w72
            frame #0 {
              n28 = control-ref of="Status"() -> (w90:refnum<vi>)
              n29 = call "Get Chan Data for typedefs.vi"("Custom Device Ref"=w86, "error in"=w87, "Ctl Ref"=w90, "Section Ref in"=w88) -> ("error out"=w91:errorcluster, "Section Ref out"=w92:T40)  [unwired: 5 in, 1 out]
              n30 = control-ref of="Config"() -> (w89:refnum<vi>)
              n31 = call "Get Chan Data for typedefs.vi"("Custom Device Ref"=w86, "error in"=w91, "Ctl Ref"=w89, "Section Ref in"=w92) -> ("error out"=w93:errorcluster)  [unwired: 5 in, 2 out]
            }
            frame #1 {
            }
          }
          n32 = Bundle By Name(cluster=w85, "FIFO Indexes.Read.HH Status"=w73, "FIFO Indexes.Write.HH Config"=w72) -> (w84:T7)
        }
        frame 2 {
          # "DI-A"
          n33 = global read "DCM Constants and GUIDs.vi" "GUID.DI (Bank A)"() -> (w123:string)
          n34 = global read "DCM Properties.vi" "DI-A.Configuration"() -> (w119:string)
          n35 = global read "DCM Constants and GUIDs.vi" "ChanList.DI Fault Clear"() -> (w125:T41[])
          n36 = global read "DCM Constants and GUIDs.vi" "Constant.Clear Faults"() -> (w124:string)
          n37 = global read "DCM Constants and GUIDs.vi" "ChanList.DI Config"() -> (w126:T41[])
          n38 = call-poly <vilib>:"NI VeriStand - Search for Item.vi"("error in"=w128, "Item GUID"=w123, "Section Ref in"=w127) -> ("error out"=w104:errorcluster, "Item Ref"=w105:T40, "Section Ref out"=w118:T40, "Found"=w106:bool)  [unwired: 5 in]
          n39 = case shown="True" w106 {
            tunnel: w119 -> [_ w139]
            tunnel: [w131 w137] -> w98
            tunnel: [w129 w134] -> w102
            tunnel: w105 -> [w130 w136]
            tunnel: w104 -> [w129 w135]
            tunnel: [w130 w133] -> w103
            tunnel: T12 {"Configuration"=enum."Solenoid Unipolar 4", "Power Supply Enable"=FALSE, "Boost Voltage [V]"=0.0, "Inject Enable"=FALSE, "DI Zener Enable"=FALSE, "DI Zener Voltage [V]"=0.0, "Pump Zener Enable"=FALSE, "Pump Zener Voltage [V]"=0.0, "Boost Clamp [V]"=0.0} ("Settings.A Configuration") -> [w131 w132]
            frame False {
            }
            frame True {
              n40 = call "Flatten and Get String Property.vi"("error in (no error)"=w135, "Default Value"=w132, "Property Name"=w139, "Section Ref in"=w136) -> ("error out"=w134:errorcluster, "Value"=w138:variant, "Section Ref out"=w133:T40)  [unwired: 5 in]
              n41 = Variant To Data(type=w132, Variant=w138) -> (data=w137:T12)  [unwired: 1 in, 1 out]
            }
          }
          n42 = control-ref of="Faults"() -> (w108:refnum<vi>)
          n43 = call "Get Chan Data for typedefs.vi"("Custom Device Ref"=w118, "error in"=w102, "Ctl Ref"=w108, "Section Ref in"=w103) -> ("error out"=w107:errorcluster, "Section Ref out"=w101:T40)  [unwired: 5 in, 1 out]
          n44 = flat-sequence {
            tunnel: w107 -> [w141]
            tunnel: [w141] -> w100
            tunnel: ["Faults"] -> w109
            frame #0 {
            }
          }
          n45 = for {
            tunnel: w126 -> [w145] mode=indexing
            tunnel: [w144] -> w117 mode=indexing
            n46 = Unbundle By Name(w145) -> ("Name"=w144:string)
          }
          n47 = for {
            tunnel: w125 -> [w143] mode=indexing
            tunnel: [w142] -> w114 mode=indexing
            n48 = Unbundle By Name(w143) -> ("Name"=w142:string)
          }
          n49 = call "Get Channel Data in Section.vi"("Custom device ref"=w118, "error in (no error)"=w100, "Channels"=w117, "Item Ref in"=w101) -> ("error out"=w116:errorcluster, "FIFO indexes"=w113:i32[], "Item Ref out"=w115:T40)  [unwired: 3 in, 2 out]
          n50 = call "Get Channel Data in Section.vi"("Custom device ref"=w118, "error in (no error)"=w116, "Channels"=w114, "Section (\"\":none)"=w124, "Item Ref in"=w115) -> ("error out"=w122:errorcluster, "FIFO indexes"=w112:i32[])  [unwired: 2 in, 3 out]
          n51 = Array To Cluster(array=w113) -> (cluster=w111:T42)
          n52 = Array To Cluster(array=w112) -> (cluster=w110:T43)
          n53 = Bundle By Name(cluster=w121, "Settings.A Configuration"=w98, "FIFO Indexes.Read.A DI Faults"=w109, "FIFO Indexes.Write.A Config"=w111, "FIFO Indexes.Write.A Fault Clear"=w110) -> (w120:T7)
        }
        frame 3 {
          # "DI-B"
          n54 = global read "DCM Constants and GUIDs.vi" "GUID.DI (Bank B)"() -> (w171:string)
          n55 = global read "DCM Properties.vi" "DI-B.Configuration"() -> (w167:string)
          n56 = global read "DCM Constants and GUIDs.vi" "ChanList.DI Fault Clear"() -> (w173:T41[])
          n57 = global read "DCM Constants and GUIDs.vi" "Constant.Clear Faults"() -> (w172:string)
          n58 = global read "DCM Constants and GUIDs.vi" "ChanList.DI Config"() -> (w174:T41[])
          n59 = call-poly <vilib>:"NI VeriStand - Search for Item.vi"("error in"=w176, "Item GUID"=w171, "Section Ref in"=w175) -> ("error out"=w151:errorcluster, "Item Ref"=w152:T40, "Section Ref out"=w166:T40, "Found"=w153:bool)  [unwired: 5 in]
          n60 = case shown="True" w153 {
            tunnel: w167 -> [_ w187]
            tunnel: [w179 w185] -> w159
            tunnel: [w177 w182] -> w149
            tunnel: w152 -> [w178 w184]
            tunnel: w151 -> [w177 w183]
            tunnel: [w178 w181] -> w150
            tunnel: T12 {"Configuration"=enum."Solenoid Unipolar 4", "Power Supply Enable"=FALSE, "Boost Voltage [V]"=0.0, "Inject Enable"=FALSE, "DI Zener Enable"=FALSE, "DI Zener Voltage [V]"=0.0, "Pump Zener Enable"=FALSE, "Pump Zener Voltage [V]"=0.0, "Boost Clamp [V]"=0.0} ("outputs.A Configuration") -> [w179 w180]
            frame False {
            }
            frame True {
              n61 = call "Flatten and Get String Property.vi"("error in (no error)"=w183, "Default Value"=w180, "Property Name"=w187, "Section Ref in"=w184) -> ("error out"=w182:errorcluster, "Value"=w186:variant, "Section Ref out"=w181:T40)  [unwired: 5 in]
              n62 = Variant To Data(type=w180, Variant=w186) -> (data=w185:T12)  [unwired: 1 in, 1 out]
            }
          }
          n63 = control-ref of="Faults"() -> (w155:refnum<vi>)
          n64 = call "Get Chan Data for typedefs.vi"("Custom Device Ref"=w166, "error in"=w149, "Ctl Ref"=w155, "Section Ref in"=w150) -> ("error out"=w154:errorcluster, "Section Ref out"=w147:T40)  [unwired: 5 in, 1 out]
          n65 = flat-sequence {
            tunnel: w154 -> [w189]
            tunnel: [w189] -> w146
            tunnel: ["Faults"] -> w156
            frame #0 {
            }
          }
          n66 = for {
            tunnel: w174 -> [w193] mode=indexing
            tunnel: [w192] -> w165 mode=indexing
            n67 = Unbundle By Name(w193) -> ("Name"=w192:string)
          }
          n68 = for {
            tunnel: w173 -> [w191] mode=indexing
            tunnel: [w190] -> w162 mode=indexing
            n69 = Unbundle By Name(w191) -> ("Name"=w190:string)
          }
          n70 = call "Get Channel Data in Section.vi"("Custom device ref"=w166, "error in (no error)"=w146, "Channels"=w165, "Item Ref in"=w147) -> ("error out"=w164:errorcluster, "FIFO indexes"=w161:i32[], "Item Ref out"=w163:T40)  [unwired: 3 in, 2 out]
          n71 = call "Get Channel Data in Section.vi"("Custom device ref"=w166, "error in (no error)"=w164, "Channels"=w162, "Section (\"\":none)"=w172, "Item Ref in"=w163) -> ("error out"=w170:errorcluster, "FIFO indexes"=w160:i32[])  [unwired: 2 in, 3 out]
          n72 = Array To Cluster(array=w161) -> (cluster=w158:T42)
          n73 = Array To Cluster(array=w160) -> (cluster=w157:T43)
          n74 = Bundle By Name(cluster=w169, "Settings.B Configuration"=w159, "FIFO Indexes.Read.B DI Faults"=w156, "FIFO Indexes.Write.B Config"=w158, "FIFO Indexes.Write.B Fault Clear"=w157) -> (w168:T7)
        }
      }
    }
    n75 = in-place-cluster #1("DCM Core"=w7) -> (→"Compiled Data":T1)
  }
  "error out" <- w3
  "Device Item Ref out" <- w4
